vi "Initialize.vi"(8 "error in (no error)":errorcluster, 11 "Agitator Module State Cluster":T1={"State"=enum."Idle", "Start Time"=timestamp(0 s since 1904-01-01), "Current Time"=timestamp(0 s since 1904-01-01), "Agitator Module Config"={"GUID"="", "Drop Coords"={"Horizontal"=0, "Vertical"=0}, "Process Name"="", "User name"="", "Queue Name"="", "Settings"={"Cycle Period"=500.0, "Agitator Type"="", "Setpoint (µm)"=0.0, "IKA EUROSTAR Settings"={"VISA resource name"="", "Simulated?"=FALSE}}, "Load Count"=0}, "Output Error"=FALSE, "Log Started"=FALSE, "First Iteration"=FALSE, "Data"={"Agitator rpm Value"=0.0}, "Agitator On?"=enum."Off"}) -> (0 "error out":errorcluster, 1 "Initialized":bool, 3 "Agitator Module State Cluster":T1={"State"=enum."Idle", "Start Time"=timestamp(0 s since 1904-01-01), "Current Time"=timestamp(0 s since 1904-01-01), "Agitator Module Config"={"GUID"="", "Drop Coords"={"Horizontal"=0, "Vertical"=0}, "Process Name"="", "User name"="", "Queue Name"="", "Settings"={"Cycle Period"=500.0, "Agitator Type"="", "Setpoint (µm)"=0.0, "IKA EUROSTAR Settings"={"VISA resource name"="", "Simulated?"=FALSE}}, "Load Count"=0}, "Output Error"=FALSE, "Log Started"=FALSE, "First Iteration"=FALSE, "Data"={"Agitator rpm Value"=0.0}, "Agitator On?"=enum."Off"})   [LabVIEW 2018, in "Agitator Module.lvlib" / "Agitator Module Engine.lvlib"]
uses:
  Agitator Module Engine.lvlib
  Feed Module/Controls/Agitator Module State Cluster.ctl
  Pump Module Folder/Measure Instrument/State Enum.ctl
  Feed Module/Controls/Agitator Module Config Cluster.ctl
  <vilib>/Utility/miscctls.llb/LVPoint32TypeDef.ctl
  Feed Module/Controls/Agitator Module Settings Cluster.ctl
  IKA EUROSTAR/IKA EUROSTAR Settings.ctl
  Tag VIs/Tag FGV Operation Enum.ctl
  Shared Variables/Dynamic Shared Variables.lvlib
  Sonic Systems P100/Sonic Systems P100.lvlib
  Agitator Module.lvlib
  Pump Module Folder/Measure Instrument/Pump Module Engine.lvlib
  IKA EUROSTAR/IKA EUROSTAR.lvlib
panel:
  # "Agitator Settings"
  # "Agitator Settings"
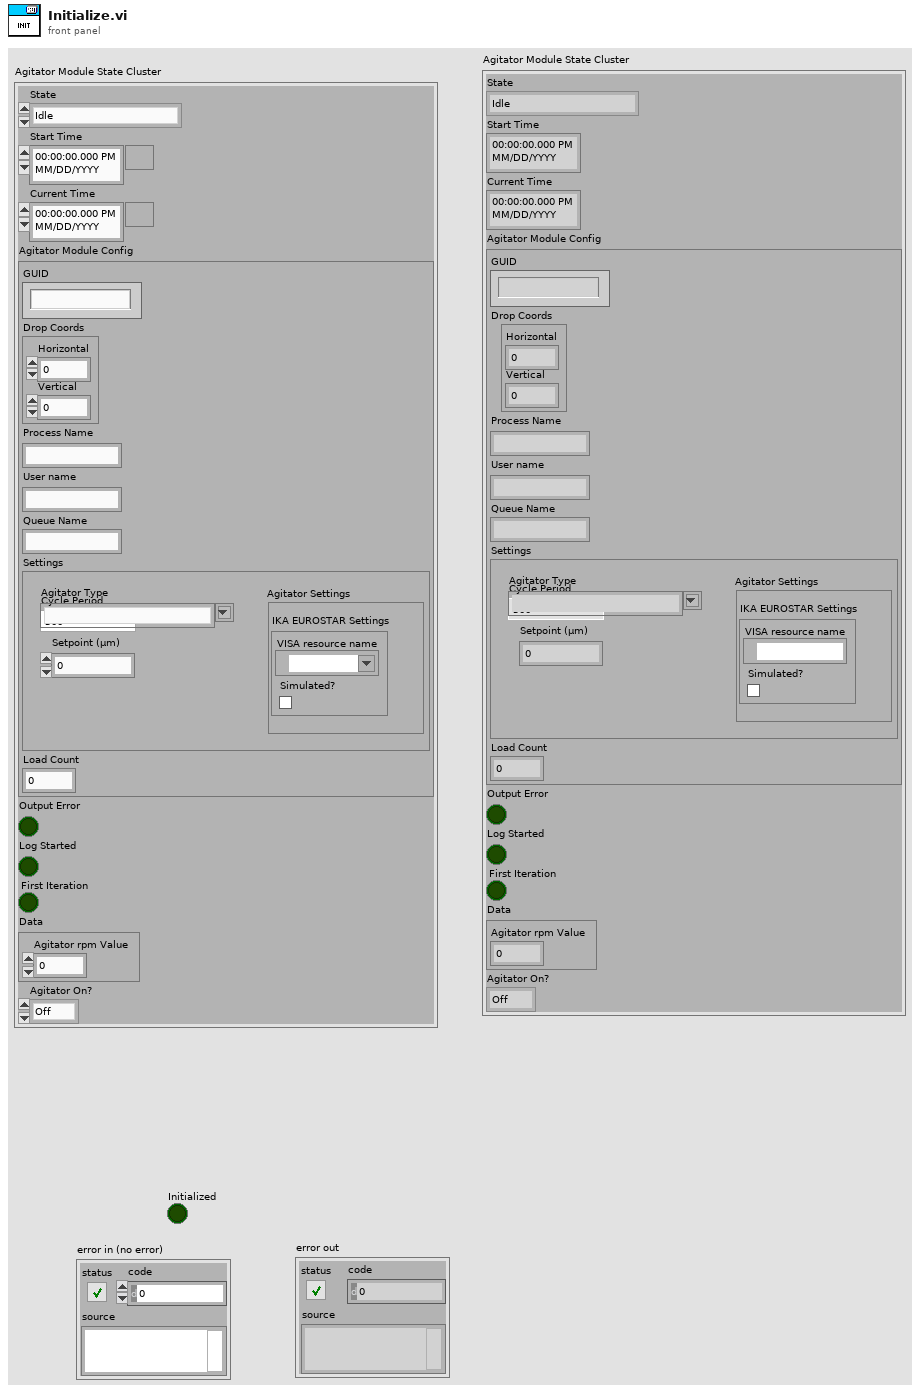
[diagram p1: front panel]
types:
  T1 = typedef "Agitator Module.lvlib/Agitator Module State Cluster.ctl" = cluster{"State":T2, "Start Time":timestamp, "Current Time":timestamp, "Agitator Module Config":T3, "Output Error":bool, "Log Started":bool, "First Iteration":bool, "Data":cluster{"Agitator rpm Value":dbl}, "Agitator On?":enum16{"Off", "On", "Not Initialized", "Over Cutoff"}}
  T2 = typedef "Pump Module.lvlib/Pump Module Engine.lvlib/State Enum.ctl" = enum16{"Measuring", "Idle", "Paused"}
  T3 = typedef "Agitator Module.lvlib/Agitator Module Config Cluster.ctl" = cluster{"GUID":string, "Drop Coords":T4, "Process Name":string, "User name":string, "Queue Name":string, "Settings":T5, "Load Count":i32}
  T4 = typedef "LVPoint32TypeDef.ctl" = cluster{"Horizontal":i32, "Vertical":i32}
  T5 = typedef "Agitator Module.lvlib/Agitator Module Settings Cluster.ctl" = cluster{"Cycle Period":dbl, "Agitator Type":string, "Setpoint (µm)":dbl, "IKA EUROSTAR Settings":T6}
  T6 = typedef "IKA EUROSTAR.lvlib/IKA EUROSTAR Settings.ctl" = cluster{"VISA resource name":refnum<visa-resource-name>, "Simulated?":bool}
  T7 = typedef "Tag FGV Operation Enum.ctl" = enum16{"Init", "Set Notification Queue", "Create Tag", "Commit", "Write Tag (Numeric)", "Write Tag (Boolean)", "Read All Tags", "Read One Tag", "Delete Tag Category", "Set Alarm Parameters (Numeric)", "Set Alarm Parameters (Boolean)", "Enable All Alarms", "Disable All Alarms", "Delete All Tags", "Read Alarms", "Ack Alarm", "Read Alarm Parameters (Numeric)", "Read Alarm Parameters (Boolean)"}
  T8 = cluster{"Amplitude Tag":string, "Power Tag":string, "Output Device Tag":string}
  T9 = typedef "Sonic Systems P100.lvlib/Sonic Systems P100 Settings.ctl" = cluster{"VISA resource name":refnum<visa-resource-name>, "Simulated?":bool}
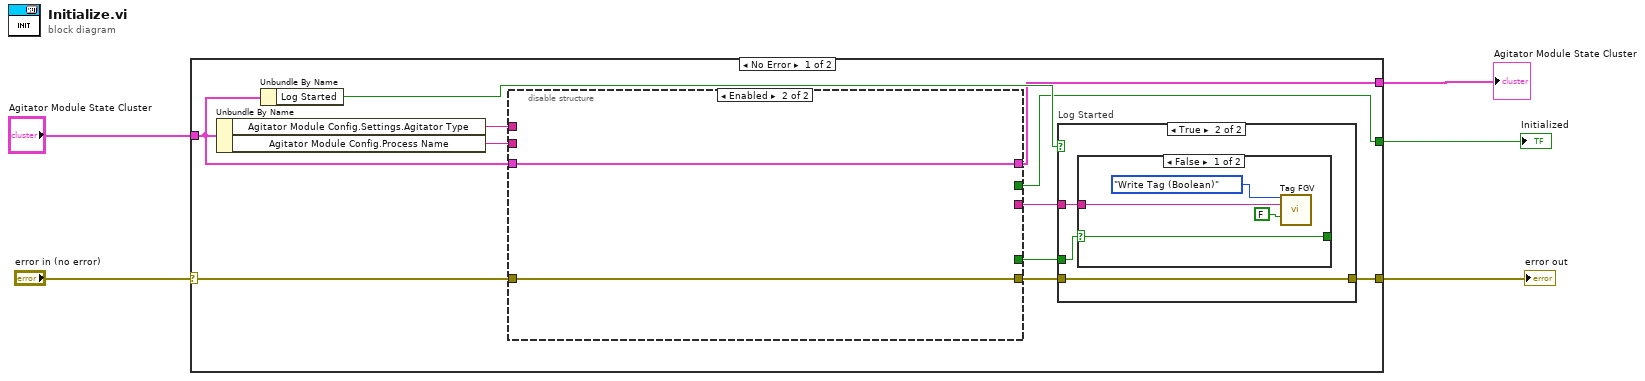
[diagram p0: block diagram]
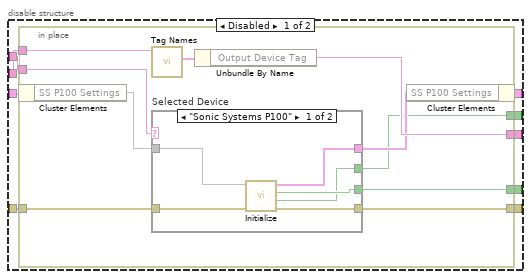
[diagram p2: hidden frame]
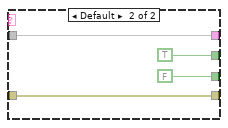
[diagram p3: hidden frame]
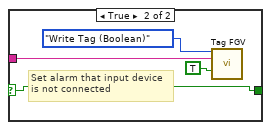
[diagram p5: hidden frame]
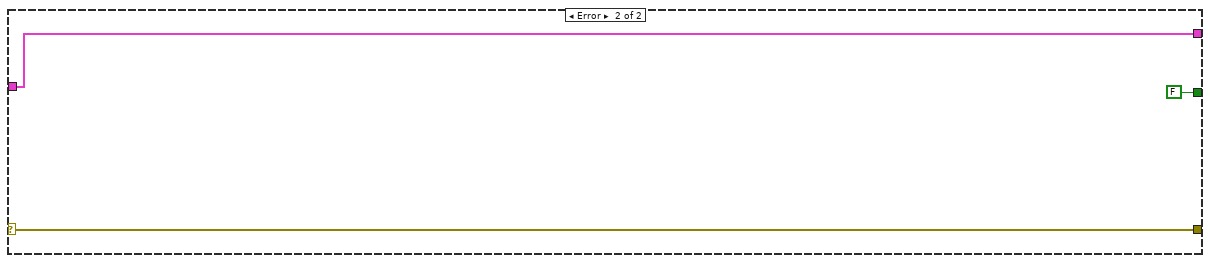
[diagram p6: hidden frame]
diagram:
  n1 = case shown="No Error" "error in (no error)" {
    selector: "error in (no error)" -> [w15 w62]
    tunnel: [w12 w62] -> w4
    tunnel: "Agitator Module State Cluster" -> [w6 w61]
    tunnel: [w9 w61] -> w2
    tunnel: [w7 FALSE ("Initialized")] -> w3
    frame No Error {
      n2 = Unbundle By Name(w6) -> ("Agitator Module Config.Settings.Agitator Type"=w16:string, "Agitator Module Config.Process Name"=w14:string)
      n3 = Unbundle By Name(w6) -> ("Log Started"=w10:bool)
      n4 = disable-structure shown="Enabled" {
        disable-tunnel: w16 -> [w25 _]
        disable-tunnel: w15 -> [w24 w46]
        disable-tunnel: w14 -> [w23 _]
        disable-tunnel: [w22 w46] -> w13
        disable-tunnel: [w21 _] -> w11
        disable-tunnel: [w20 w47] -> w9
        disable-tunnel: [w19 _] -> w8
        disable-tunnel: [w18 _] -> w7
        disable-tunnel: w6 -> [w17 w47]
        frame Disabled {
          n5 = in-place {
            in-place-border: w25 -> [w35]
            in-place-border: w24 -> [w34]
            in-place-border: w23 -> [w33]
            in-place-border: [w32] -> w22
            in-place-border: [w30] -> w21
            in-place-border: [w27] -> w19
            in-place-border: [w26] -> w18
            n6 = in-place-cluster #1(w17) -> ("SS P100 Settings"=w29)
            n7 = call "Tag Names.vi"("Process Name"=w33) -> ("SC Tags"=w31:T8)  [unwired: 8 in, 2 out]
            n8 = case "Selected Device" shown="\"Sonic Systems P100\"" w35 {
              tunnel: w29 -> [w41 w45]
              tunnel: w34 -> [w40 w44]
              tunnel: [w38 w44] -> w32
              tunnel: [w39 w45] -> w28
              tunnel: [w37 FALSE ("Connection Error")] -> w27
              tunnel: [w36 TRUE ("Initialized")] -> w26
              frame "Sonic Systems P100" {
                n9 = call "Initialize.vi"("error in (no error)"=w40, "SS P100 Settings"=w41) -> ("error out"=w38:errorcluster, "Initialized"=w36:bool, "Connection Error"=w37:bool, "SS P100 Settings"=w39:T9)  [unwired: 6 in]
              }
              frame Default {
              }
            }
            n10 = Unbundle By Name(w31) -> ("Output Device Tag"=w30:string)
            n11 = in-place-cluster #1("SS P100 Settings"=w28) -> (w20:T1)
          }
        }
        frame Enabled {
        }
      }
      n12 = case "Log Started" shown="True" w10 {
        tunnel: w13 -> [w48 w49]
        tunnel: [w48 w49] -> w12
        tunnel: w11 -> [_ w51]
        tunnel: w8 -> [_ w50]
        frame False {
        }
        frame True {
          n13 = case shown="False" w50 {
            selector: w50 -> [w55 w59]
            tunnel: [w55 w59] -> _
            tunnel: w51 -> [w53 w57]
            frame False {
              n14 = call "Tag FGV.vi"("Operation"=Tag_FGV_Operation_Enum."Write Tag (Boolean)", "Tag Name"=w53, "Data"=FALSE) -> ()  [unwired: 5 in, 8 out]
            }
            frame True {
              # "Set alarm that input device\nis not connected"
              n15 = call "Tag FGV.vi"("Operation"=Tag_FGV_Operation_Enum."Write Tag (Boolean)", "Tag Name"=w57, "Data"=TRUE) -> ()  [unwired: 5 in, 8 out]
            }
          }
        }
      }
    }
    frame Error {
    }
  }
  "error out" <- w4
  "Initialized" <- w3
  "Agitator Module State Cluster" <- w2
